vi "interpolate 1d linear.vi"(9 "xi":dbl[](array[numeric]), 10 "Y":dbl[](array[numeric]), 11 "X":dbl[](array[numeric])) -> (3 "yi":dbl[](array[numeric]))   [LabVIEW 2021, in "RocketPlot.lvlib"]
uses:
  RocketPlot.lvlib
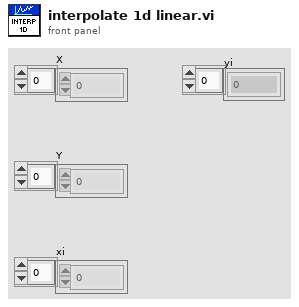
[diagram p1: front panel]
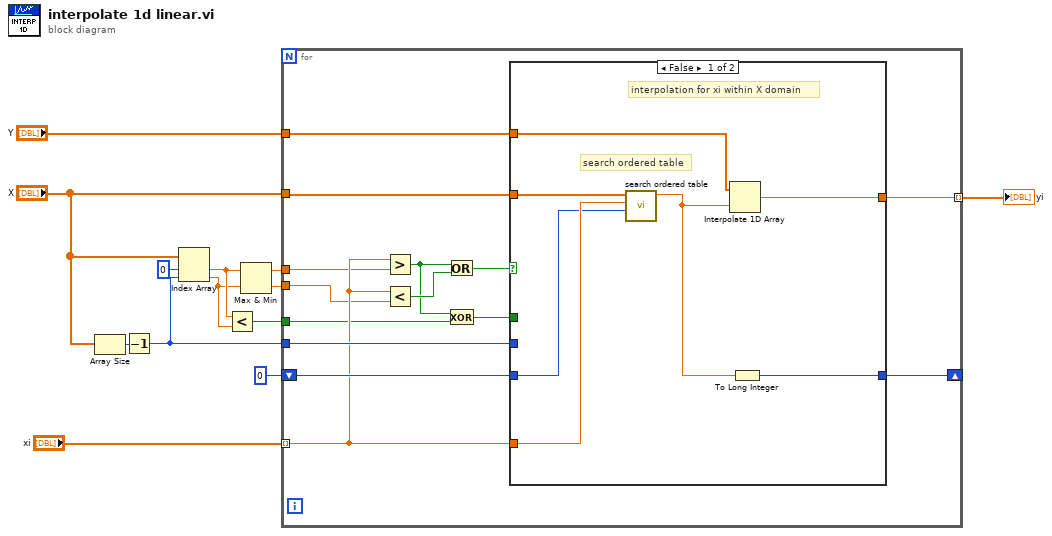
[diagram p0: block diagram]
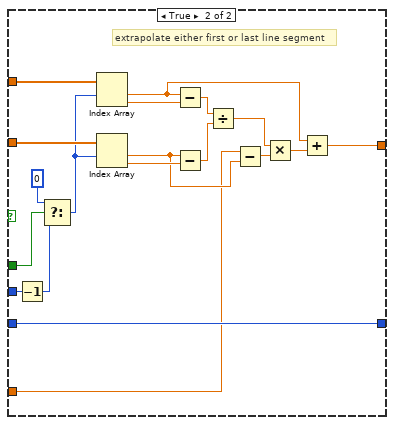
[diagram p2: hidden frame]
diagram:
  n1 = Array Size(array="X") -> (size(s)=w8:i32)
  n2 = Decrement(x=w8) -> (x-1=w7:i32)
  n3 = Index Array(array="X", index #1=0 ("index"), index #2=w7) -> (element #1=w4:dbl, element #2=w3:dbl)
  n4 = Less?(x=w4, y=w3) -> (x < y?=w5:bool)
  n5 = Max & Min(x=w4, y=w3) -> (max(x,y)=w2:dbl, min(x,y)=w1:dbl)
  n6 = for {
    tunnel: "X" -> [w27]
    tunnel: "Y" -> [w26]
    tunnel: [w25] -> w11 mode=indexing
    tunnel: w1 -> [w14]
    tunnel: w2 -> [w15]
    tunnel: w7 -> [w23]
    shift-right: [w21] -> _
    shift-left: 0 ("index") -> [w22]
    tunnel: "xi" -> [w20] mode=indexing
    tunnel: w5 -> [w19]
    n7 = Greater?(x=w20, y=w15) -> (0:w16:bool)
    n8 = Less?(x=w20, y=w14) -> (x < y?=w18:bool)
    n9 = Or(x=w16, y=w18) -> (x .or. y?=w24:bool)
    n10 = Exclusive Or(1:w19, 2:w16) -> (0:w17:bool)
    n11 = case shown="False" w24 {
      tunnel: w27 -> [w30 w53]
      tunnel: w26 -> [w34 w52]
      tunnel: [w33 w51] -> w25
      tunnel: w17 -> [_ w39]
      tunnel: w23 -> [_ w50]
      tunnel: w22 -> [w28 w36]
      tunnel: [w32 w36] -> w21
      tunnel: w20 -> [w29 w35]
      frame False {
        # "search ordered table"
        # "interpolation for xi within X domain"
        n12 = call "search ordered table.vi"("starting index"=w28, "x value"=w29, "ordered x array"=w30) -> ("fractional index"=w31:dbl)  [unwired: 8 in]
        n13 = Interpolate 1D Array(1:w31, 2:w34) -> (0:w33:dbl)
        n14 = To Long Integer(number=w31) -> (32bit integer=w32:i32)
      }
      frame True {
        # "extrapolate either first or last line segment"
        n15 = Decrement(x=w50) -> (x-1=w40:i32)
        n16 = Select(t=0, s=w39, f=w40) -> (s? t:f=w37:i32)
        n17 = Index Array(array=w52, index #1=w37) -> (element #1=w47:dbl, element #2=w49:dbl)  [unwired: 1 in]
        n18 = Index Array(array=w53, index #1=w37) -> (element #1=w46:dbl, element #2=w48:dbl)  [unwired: 1 in]
        n19 = Subtract(x=w47, y=w49) -> (x-y=w45:dbl)
        n20 = Subtract(x=w46, y=w48) -> (x-y=w44:dbl)
        n21 = Divide(x=w45, y=w44) -> (x/y=w42:dbl)
        n22 = Subtract(x=w35, y=w46) -> (x-y=w43:dbl)
        n23 = Multiply(x=w42, y=w43) -> (x*y=w41:dbl)
        n24 = Add(x=w47, y=w41) -> (x+y=w51:dbl)
      }
    }
  }
  "yi" <- w11
